vi "isBehind.vi"() -> ()   [LabVIEW 2009]
panel:
  in  "Line Angle":dbl
  in  "Landmark Relative Location":cluster{"x":dbl, "y":dbl}
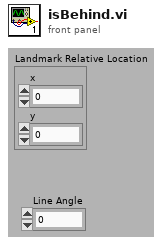
[diagram p1: front panel]
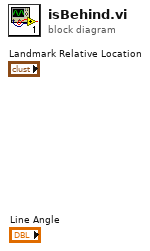
[diagram p0: block diagram]
diagram:
